vi "Filter Application Components.vi"() -> ()   [LabVIEW 2020, in "PicoG-Processor.lvlib" / "WebProjectWatcher.lvclass"]
uses:
  WebProjectWatcher.lvclass
panel:
  out "Vireo Component Ids":string[](array[string])
  out "error out":errorcluster
  in  "error in (no error)":errorcluster
  in  "Vireo Target ID":string
  out "XML":refnum<k20>
  in  "XML in":refnum<k20>
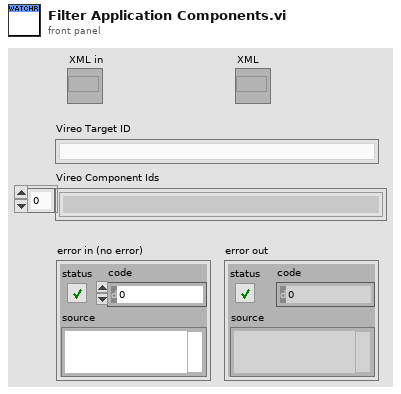
[diagram p1: front panel]
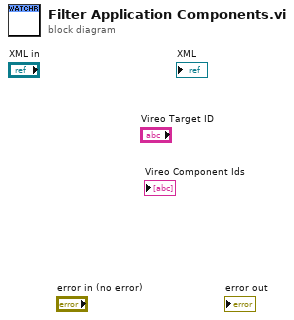
[diagram p0: block diagram]
diagram:
